vi "SetOutputFreq.vi"(8 "error in (no error)":errorcluster, 9 "Output enabled":bool=TRUE, 10 "Output mixer fequency [MHz]":dbl, 11 "Scope5785_six_channel":refnum<class "Scope5782_six_channel.lvclass">) -> (0 "error out":errorcluster, 3 "Scope5785_six_channel out":refnum<class "Scope5782_six_channel.lvclass">)   [LabVIEW 2018, in "Scope5782_six_channel.lvclass"]
uses:
  Scope5782_six_channel.lvclass
  Scope5782_six_channel.lvclass/Scope5782_six_channel.ctl
  FpgaRef/FpgaRef5782/FpgaRef5782.lvclass
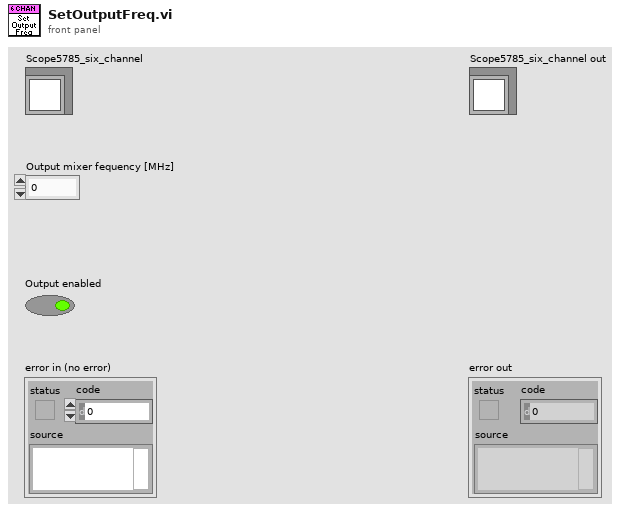
[diagram p1: front panel]
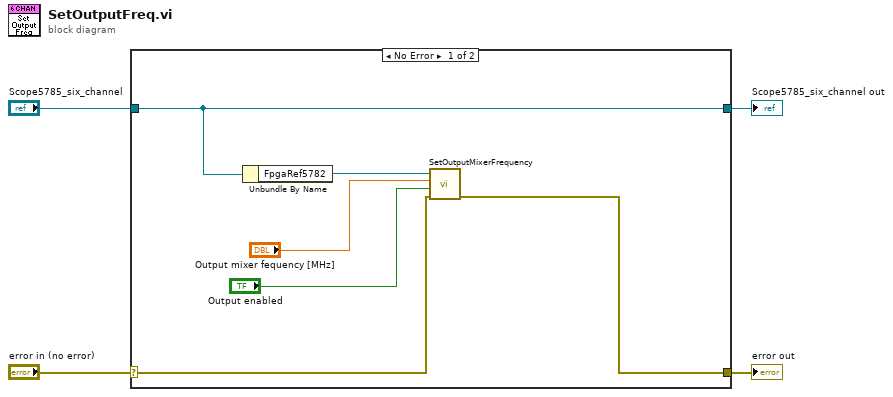
[diagram p0: block diagram]
diagram:
  n1 = case shown="No Error" "error in (no error)" {
    selector: "error in (no error)" -> [w6 w12]
    tunnel: [w5 w12] -> w3
    tunnel: [w10 w11] -> w1
    tunnel: "Scope5785_six_channel" -> [w10 w11]
    frame No Error {
      n2 = Unbundle By Name(w10) -> ("FpgaRef5782"=w9:refnum<class "FpgaRef5782.lvclass">)
      n3 = call "SetOutputMixerFrequency.vi"("error in (no error)"=w6, "Output enabled"="Output enabled", "Output mixer fequency [MHz]"="Output mixer fequency [MHz]", "FpgaRef5782 in"=w9) -> ("error out"=w5:errorcluster)  [unwired: 6 in, 1 out]
    }
    frame Error {
    }
  }
  "error out" <- w3
  "Scope5785_six_channel out" <- w1
